vi "simple approval test.vi"() -> ()   [LabVIEW 2020]
uses:
  <vilib>/addons/_JKI Toolkits/Caraya/classes/Assert/Assert True.vi
  <vilib>/addons/_JKI Toolkits/Caraya/classes/Test/Test.lvclass
  <vilib>/addons/_JKI Toolkits/Caraya/classes/Assert/Assert.lvclass
  Approval Tests/Approval Tests.lvlib
panel:
  out "Failure Message":string
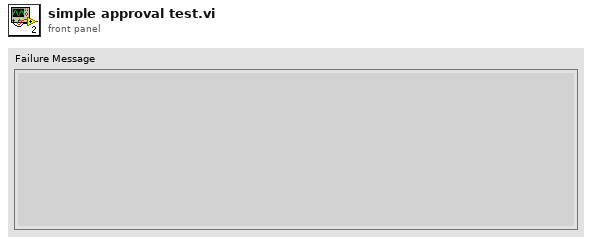
[diagram p1: front panel]
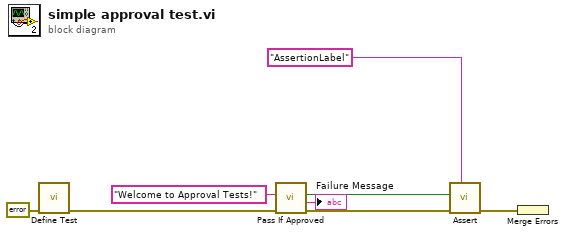
[diagram p0: block diagram]
diagram:
  n1 = call <vilib>:"Define Test.vi"("error in (no error)"=errorcluster {"status"=FALSE, "code"=0, "source"=""}) -> ("error out"=w5:errorcluster)  [unwired: 9 in, 1 out]
  n2 = call "Pass If Approved.vi"("error in"=w5, "Test Data"="Welcome to Approval Tests!") -> ("error out"=w4:errorcluster, "Failure Message"=→"Failure Message":string, "Passed?"=w2:bool)  [unwired: 7 in]
  n3 = call-poly <vilib>:"Assert.vi"("Label"="AssertionLabel" ("Label (VI Title)"), "error in (no error)"=w4, "True?"=w2) -> ("error out"=w7:errorcluster)  [unwired: 7 in, 1 out]
  n4 = Merge Errors(w7) -> ()  [unwired: 1 out]
